vi "Stop Laser.vi"(8 "error in (no error)":errorcluster, 11 "Laser API in":refnum<class "Laser API.lvclass">) -> (0 "error out":errorcluster, 3 "Laser API out":refnum<class "Laser API.lvclass">)   [LabVIEW 2022 SP3, in "Laser API.lvclass"]
uses:
  Laser API.lvclass
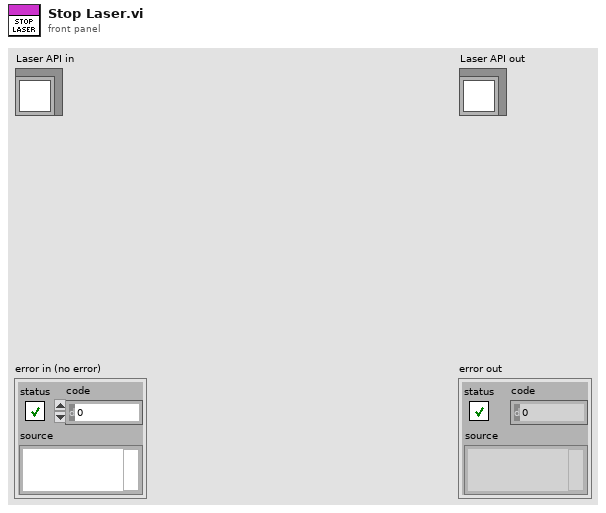
[diagram p1: front panel]
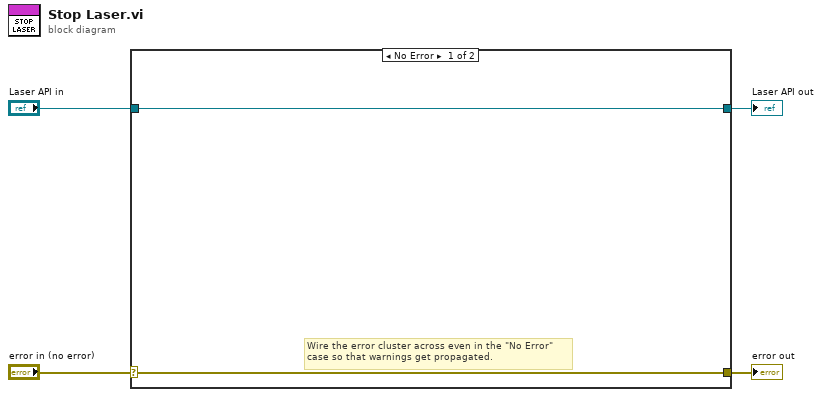
[diagram p0: block diagram]
diagram:
  n1 = case shown="No Error" "error in (no error)" {
    selector: "error in (no error)" -> [w5 w8]
    tunnel: [w5 w8] -> w3
    tunnel: [w6 w7] -> w1
    tunnel: "Laser API in" -> [w6 w7]
    frame No Error {
      # "Wire the error cluster across even in the \"No Error\"\ncase so that warnings get propagated."
    }
    frame Error {
    }
  }
  "error out" <- w3
  "Laser API out" <- w1
